vi "motor_2.vi"(7 "dt (s)":dbl=-1.0 format="%.3f", 8 "error in (no error)":errorcluster, 9 "PID gains":T1, 10 "Last Position":dbl[](array[numeric]), 11 "Input Pulse Per Sec":dbl[](array[numeric])) -> (0 "error out":errorcluster, 2 "Current Position":i32[](array[numeric]), 3 "Current Speed":i32[](array[numeric]))   [LabVIEW 2016]
uses:
  <vilib>/myRIO/Common/Instrument Driver Framework/myRIO v1.0/Encoder/typedefs/Encoder Signal Mode.ctl
  <vilib>/myRIO/Instrument Drivers/Onboard IO/Encoder/typedefs/Encoder Reference.ctl
  <vilib>/myRIO/Common/Instrument Driver Framework/Utilities/typedefs/myRIO Generic Hardware Reference.ctl
  <vilib>/myRIO/Common/Instrument Driver Framework/Utilities/typedefs/Hardware Version Enum.ctl
  <vilib>/myRIO/Common/Instrument Driver Framework/Utilities/typedefs/myRIO v1.0 Reference.ctl
  <vilib>/myRIO/Common/Instrument Driver Framework/Utilities/typedefs/Generic FPGA Reference.ctl
  <vilib>/myRIO/Common/Instrument Driver Framework/myRIO v1.0/Encoder/typedefs/Encoder Channels Enum.ctl
  <vilib>/myRIO/Common/Instrument Driver Framework/myRIO v1.0/Encoder/typedefs/Encoder Configuration v1.0.ctl
  <vilib>/userdefined/High Color/nirio_resource_hc.ctl
  <vilib>/myRIO/Instrument Drivers/Onboard IO/PWM/typedefs/PWM Reference.ctl
  <vilib>/myRIO/Common/Instrument Driver Framework/myRIO v1.0/PWM/typedefs/PWM Channels Enum.ctl
  <vilib>/myRIO/Instrument Drivers/Onboard IO/PWM/typedefs/PWM Configuration.ctl
  <vilib>/myRIO/Instrument Drivers/Onboard IO/DIO/typedefs/DIO Reference.ctl
  <vilib>/myRIO/Common/Instrument Driver Framework/myRIO v1.0/DIO/typedefs/DIO Channels List.ctl
  <vilib>/myRIO/Common/Instrument Driver Framework/myRIO v1.0/DIO/typedefs/DIO Channels Enum.ctl
  <vilib>/myRIO/Common/Instrument Driver Framework/Utilities/vis/Is FPGA Ref Available.vi
  <vilib>/myRIO/Common/Instrument Driver Framework/myRIO v1.0/Encoder/vis/myRIO v1.1 Open Encoder.vi
  <vilib>/myRIO/Instrument Drivers/Onboard IO/Encoder/vis/Read.vi
  <vilib>/myRIO/Common/Instrument Driver Framework/myRIO v1.0/PWM/vis/myRIO v1.1 Open PWM.vi
  <vilib>/myRIO/Instrument Drivers/Onboard IO/PWM/vis/Set Duty Cycle and Frequency.vi
  <vilib>/myRIO/Common/Instrument Driver Framework/myRIO v1.0/DIO/vis/myRIO v1.1 Open DIO.vi
  <vilib>/myRIO/Instrument Drivers/Onboard IO/DIO/vis/Write.vi
  <vilib>/myRIO/Common/Instrument Driver Framework/Utilities/vis/Validate Channels.vi
  <vilib>/myRIO/Common/Instrument Driver Framework/myRIO v1.0/Encoder/vis/myRIO v1.0 Reserve Encoder.vi
  <vilib>/myRIO/Common/Instrument Driver Framework/myRIO v1.0/PWM/vis/myRIO v1.0 Reserve PWM.vi
  <vilib>/myRIO/Common/Instrument Driver Framework/myRIO v1.0/DIO/vis/myRIO v1.0 Reserve DIO.vi
  <vilib>/myRIO/Common/Instrument Driver Framework/myRIO v1.0/Encoder/vis/myRIO v1.0 Build MUX Configuration Encoder.vi
  <vilib>/myRIO/Common/Instrument Driver Framework/myRIO v1.0/Resource Manager/vis/myRIO v1.0 Reserve Channel List.vi
  <vilib>/myRIO/Common/Instrument Driver Framework/myRIO v1.0/PWM/vis/myRIO v1.0 Build MUX Configuration PWM.vi
  <vilib>/myRIO/Common/Instrument Driver Framework/myRIO v1.0/DIO/vis/myRIO v1.0 Build MUX Configuration DIO.vi
  <vilib>/myRIO/Common/Instrument Driver Framework/myRIO v1.0/Resource Manager/vis/myRIO v1.0 Create Configuration List.vi
  <vilib>/myRIO/Common/Instrument Driver Framework/myRIO v1.0/Resource Manager/vis/myRIO v1.0 Reserve Channel.vi
  <vilib>/myRIO/Common/Instrument Driver Framework/myRIO v1.0/Resource Manager/vis/myRIO v1.0 Unreserve Channel.vi
  <vilib>/myRIO/Common/Instrument Driver Framework/myRIO v1.0/Resource Manager/vis/myRIO v1.0 Build Mutex Name.vi
  <vilib>/Utility/VariantDataType/GetNumericInfo.vi
  <vilib>/Utility/error.llb/Error Cluster From Error Code.vi
  <vilib>/myRIO/Common/Instrument Driver Framework/myRIO v1.0/myRIO v1.1 Open.vi
  <vilib>/myRIO/Common/Instrument Driver Framework/Utilities/vis/IO Manager.vi
  <vilib>/myRIO/Common/Instrument Driver Framework/Utilities/vis/Configuration Manager.vi
  <vilib>/myRIO/Common/Instrument Driver Framework/myRIO v1.0/Resource Manager/vis/myRIO v1.0 Configure IO.vi
  <vilib>/myRIO/Common/Instrument Driver Framework/myRIO v1.0/myRIO v1.0 Close.vi
  <vilib>/myRIO/Common/Instrument Driver Framework/myRIO v1.0/Encoder/vis/myRIO v1.0 Configure Encoder.vi
  <vilib>/myRIO/Common/Instrument Driver Framework/myRIO v1.0/Encoder/vis/myRIO v1.0 Read Encoder.vi
  <vilib>/myRIO/Common/Instrument Driver Framework/myRIO v1.0/PWM/vis/myRIO v1.0 Write PWM.vi
  <vilib>/myRIO/Common/Instrument Driver Framework/myRIO v1.0/DIO/vis/myRIO v1.0 Write DIO.vi
  <vilib>/myRIO/Express VI/Onboard IO/Encoder/Encoder Express VI.xnode
  <vilib>/myRIO/Instrument Drivers/Onboard IO/Encoder/vis/myRIO Encoder Open.xnode
  <vilib>/myRIO/Common/Instrument Driver Framework/myRIO v1.0/Encoder/typedefs/Encoder Count Direction Enum.ctl
  <vilib>/myRIO/Express VI/Onboard IO/PWM/PWM Express VI.xnode
  <vilib>/myRIO/Instrument Drivers/Onboard IO/PWM/vis/myRIO PWM Open.xnode
  <vilib>/myRIO/Express VI/Onboard IO/DO/DO Express VI.xnode
  <vilib>/myRIO/Instrument Drivers/Onboard IO/DIO/vis/myRIO DIO Open.xnode
  <vilib>/myRIO/Instrument Drivers/Onboard IO/Encoder/Encoder.lvlib
  <vilib>/myRIO/Instrument Drivers/Onboard IO/PWM/PWM.lvlib
  <vilib>/myRIO/Instrument Drivers/Onboard IO/DIO/DIO.lvlib
panel:
  out "appended array":bool[](array[boolean])
  out "PID Signal":dbl[](array[numeric])
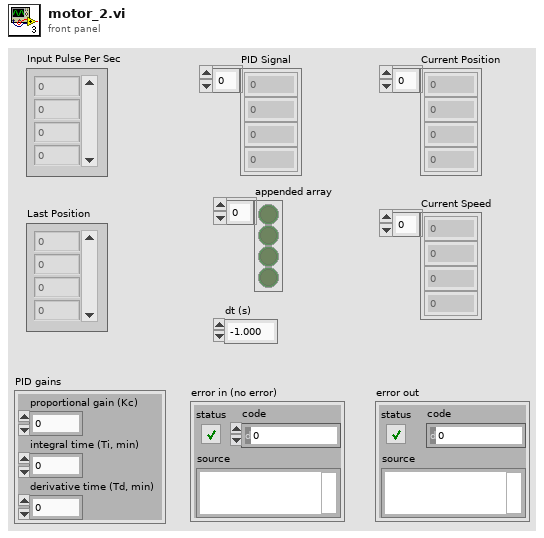
[diagram p1: front panel]
types:
  T1 = cluster{"proportional gain (Kc)":dbl, "integral time (Ti, min)":dbl, "derivative time (Td, min)":dbl}
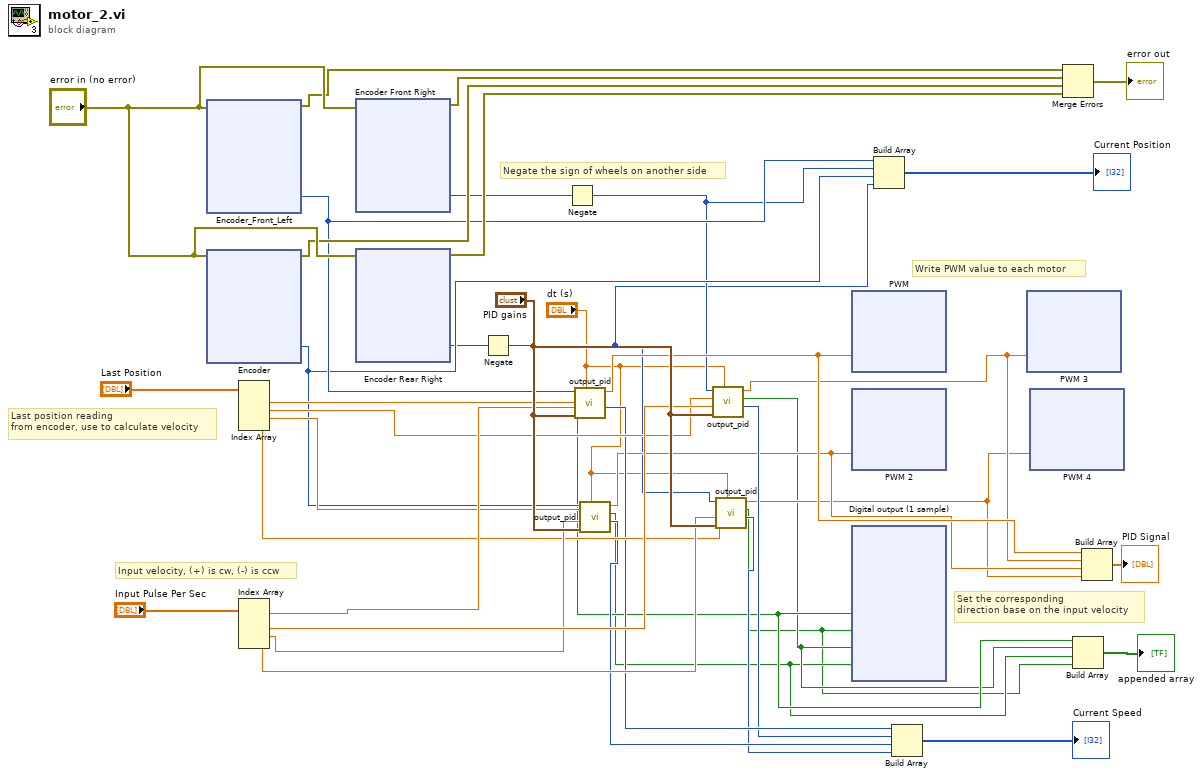
[diagram p0: block diagram]
diagram:
  # "Last position reading\nfrom encoder, use to calculate velocity"
  # "Input velocity, (+) is cw, (-) is ccw"
  # "Set the corresponding \ndirection base on the input velocity"
  # "Write PWM value to each motor"
  # "Negate the sign of wheels on another side"
  n1 = xnode "Encoder_Front_Left"("error in (no error)"="error in (no error)") -> ("Counter Value"=w24:i32, "error out"=w38:errorcluster)  [unwired: 1 in, 2 out]
  n2 = xnode "Encoder"("error in (no error)"="error in (no error)") -> ("Counter Value"=w21:i32, "error out"=w37:errorcluster)  [unwired: 1 in, 2 out]
  n3 = Index Array(array="Last Position") -> (element #1=w22:dbl, element #2=w27:dbl, element #3=w26:dbl, element #4=w25:dbl)  [unwired: 4 in]
  n4 = Index Array(array="Input Pulse Per Sec") -> (element #1=w32:dbl, element #2=w31:dbl, element #3=w30:dbl, element #4=w29:dbl)  [unwired: 4 in]
  n5 = xnode "Encoder Front Right"("error in (no error)"="error in (no error)") -> ("Counter Value"=w23:i32, "error out"=w39:errorcluster)  [unwired: 1 in, 2 out]
  n6 = xnode "Encoder Rear Right"("error in (no error)"="error in (no error)") -> ("Counter Value"=w20:i32, "error out"=w36:errorcluster)  [unwired: 1 in, 2 out]
  n7 = Negate(x=w20) -> (-x=w2:i32)
  n8 = Negate(x=w23) -> (-x=w3:i32)
  n9 = call "output_pid.vi"("dt (s)"="dt (s)", "PID gains"="PID gains", "Input Pulse Per Sec"=w32, "Last Position"=w22, "Current Position"=w24) -> ("Current Speed"=w18:i32, "DIR"=w8:bool, "PWM Signal"=w13:dbl)  [unwired: 4 in]
  n10 = call "output_pid.vi"("dt (s)"="dt (s)", "PID gains"="PID gains", "Input Pulse Per Sec"=w30, "Last Position"=w26, "Current Position"=w21) -> ("Current Speed"=w16:i32, "DIR"=w5:bool, "PWM Signal"=w11:dbl)  [unwired: 4 in]
  n11 = call "output_pid.vi"("dt (s)"="dt (s)", "PID gains"="PID gains", "Input Pulse Per Sec"=w31, "Last Position"=w27, "Current Position"=w3) -> ("Current Speed"=w17:i32, "DIR"=w6:bool, "PWM Signal"=w12:dbl)  [unwired: 4 in]
  n12 = call "output_pid.vi"("dt (s)"="dt (s)", "PID gains"="PID gains", "Input Pulse Per Sec"=w29, "Last Position"=w25, "Current Position"=w2) -> ("Current Speed"=w15:i32, "DIR"=w4:bool, "PWM Signal"=w10:dbl)  [unwired: 4 in]
  n13 = xnode "PWM"("Duty Cycle"=w13) -> ()  [unwired: 1 in, 1 out]
  n14 = xnode "PWM 2"("Duty Cycle"=w11) -> ()  [unwired: 1 in, 1 out]
  n15 = xnode "Digital output (1 sample)"("front left (A/DIO4 (Pin 19))"=w8, "rear right (B/DIO13 (Pin 26))"=w4, "front right (A/DIO13 (Pin 26))"=w6, "rear left (B/DIO4 (Pin 19))"=w5) -> ()  [unwired: 1 in, 1 out]
  n16 = Build Array(w24, w3, w21, w2) -> (→"Current Position":i32[])
  n17 = Build Array(w18, w17, w16, w15) -> (→"Current Speed":i32[])
  n18 = xnode "PWM 3"("Duty Cycle"=w12) -> ()  [unwired: 1 in, 1 out]
  n19 = xnode "PWM 4"("Duty Cycle"=w10) -> ()  [unwired: 1 in, 1 out]
  n20 = Merge Errors(w38, w39, w37, w36) -> (→"error out":errorcluster)
  n21 = Build Array(w8, w6, w5, w4) -> (→"appended array":bool[])
  n22 = Build Array(w13, w12, w11, w10) -> (→"PID Signal":dbl[])
